vi "Add_Two.vi"(9 "Numeric 2":dbl, 10 "Numeric 1":dbl) -> (2 "Add":dbl)   [LabVIEW 2018]
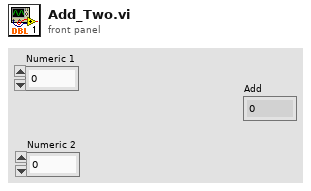
[diagram p1: front panel]
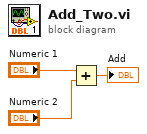
[diagram p0: block diagram]
diagram:
  n1 = Add(x="Numeric 1", y="Numeric 2") -> (x+y=→"Add":dbl)
